vi "Number Table.vi"() -> ()   [LabVIEW 2020]
panel:
  out "Array":dbl[](array[numeric]) format="%#_13g"
  in  "Numeric":dbl format="%#_13g"
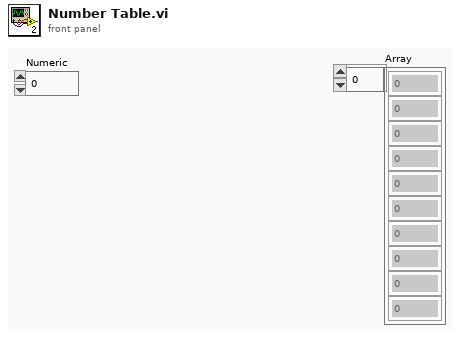
[diagram p1: front panel]
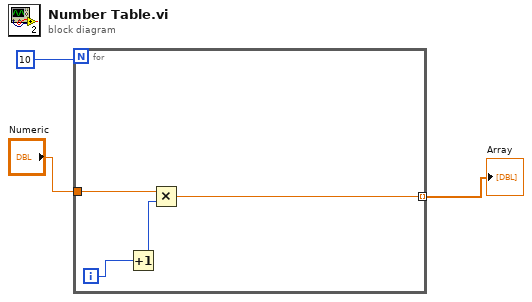
[diagram p0: block diagram]
diagram:
  n1 = for {
    N: 10 -> [_]
    tunnel: "Numeric" -> [w6]
    tunnel: [w4] -> w1 mode=indexing
    i -> [w7]
    n2 = Increment(x=w7) -> (x+1=w5:i32)
    n3 = Multiply(x=w6, y=w5) -> (x*y=w4:dbl)
  }
  "Array" <- w1
